vi "AMI1700eth_meas_he_lev.vi"(8 "error in":errorcluster, 11 "conn_id_in":refnum<k5>) -> (0 "error out":errorcluster, 2 "level":dbl, 3 "conn_id_out":refnum<k5>, 4 "status":bool)   [LabVIEW 2019]
panel:
  out "string 2":string
  out "string 1":string
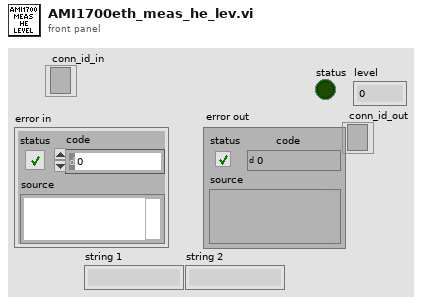
[diagram p1: front panel]
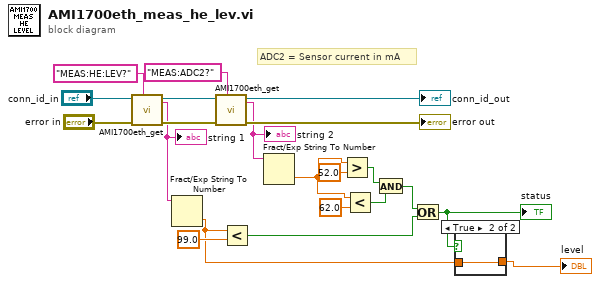
[diagram p0: block diagram]
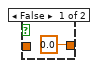
[diagram p2: hidden frame]
diagram:
  # "ADC2 = Sensor current in mA"
  n1 = call "AMI1700eth_get.vi"("command"="MEAS:HE:LEV?" ("string"), "error in"="error in", "conn_id_in"="conn_id_in") -> ("error out"=w19:errorcluster, "conn_id_out"=w20:refnum<k5>, "string"=w10:string)  [unwired: 5 in, 1 out]
  "string 1" <- w10
  n2 = Fract/Exp String To Number(string=w10) -> (number=w6:dbl)  [unwired: 3 in, 1 out]
  n3 = call "AMI1700eth_get.vi"("command"="MEAS:ADC2?" ("string"), "error in"=w19, "conn_id_in"=w20) -> ("error out"=→"error out":errorcluster, "conn_id_out"=→"conn_id_out":refnum<k5>, "string"=w17:string)  [unwired: 5 in, 1 out]
  "string 2" <- w17
  n4 = Less?(x=w6, y=99.0) -> (x < y?=w8:bool)
  n5 = Fract/Exp String To Number(string=w17) -> (number=w12:dbl)  [unwired: 3 in, 1 out]
  n6 = Greater?(x=w12, y=52.0) -> (0:w14:bool)
  n7 = Less?(x=w12, y=62.0) -> (x < y?=w13:bool)
  n8 = And(x=w14, y=w13) -> (x .and. y?=w9:bool)
  n9 = Or(x=w9, y=w8) -> (x .or. y?=w7:bool)
  "status" <- w7
  n10 = case shown="True" w7 {
    tunnel: [0.0 w23] -> w5
    tunnel: w6 -> [_ w23]
    frame False {
    }
    frame True {
    }
  }
  "level" <- w5
